vi "_interfacebrowser Build Status Menu.vi"(5 "Tree":refnum<vi>, 7 "CtlRef":refnum<vi>, 9 "Coords":T1, 11 "Menu in":refnum<k9>) -> (3 "Discard?":bool)   [LabVIEW 2017, in "interfacebrowser.lvlib"]
uses:
  interfacebrowser.lvlib
  <vilib>/Utility/miscctls.llb/LVPoint32TypeDef.ctl
  _csmHelper/API with lvcsm Support/CSM-Helper API with lvcsm Support.lvlib
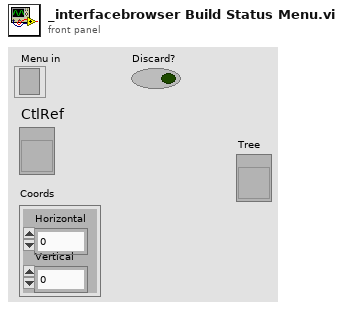
[diagram p1: front panel]
types:
  T1 = typedef "LVPoint32TypeDef.ctl" = cluster{"Horizontal":i32, "Vertical":i32}
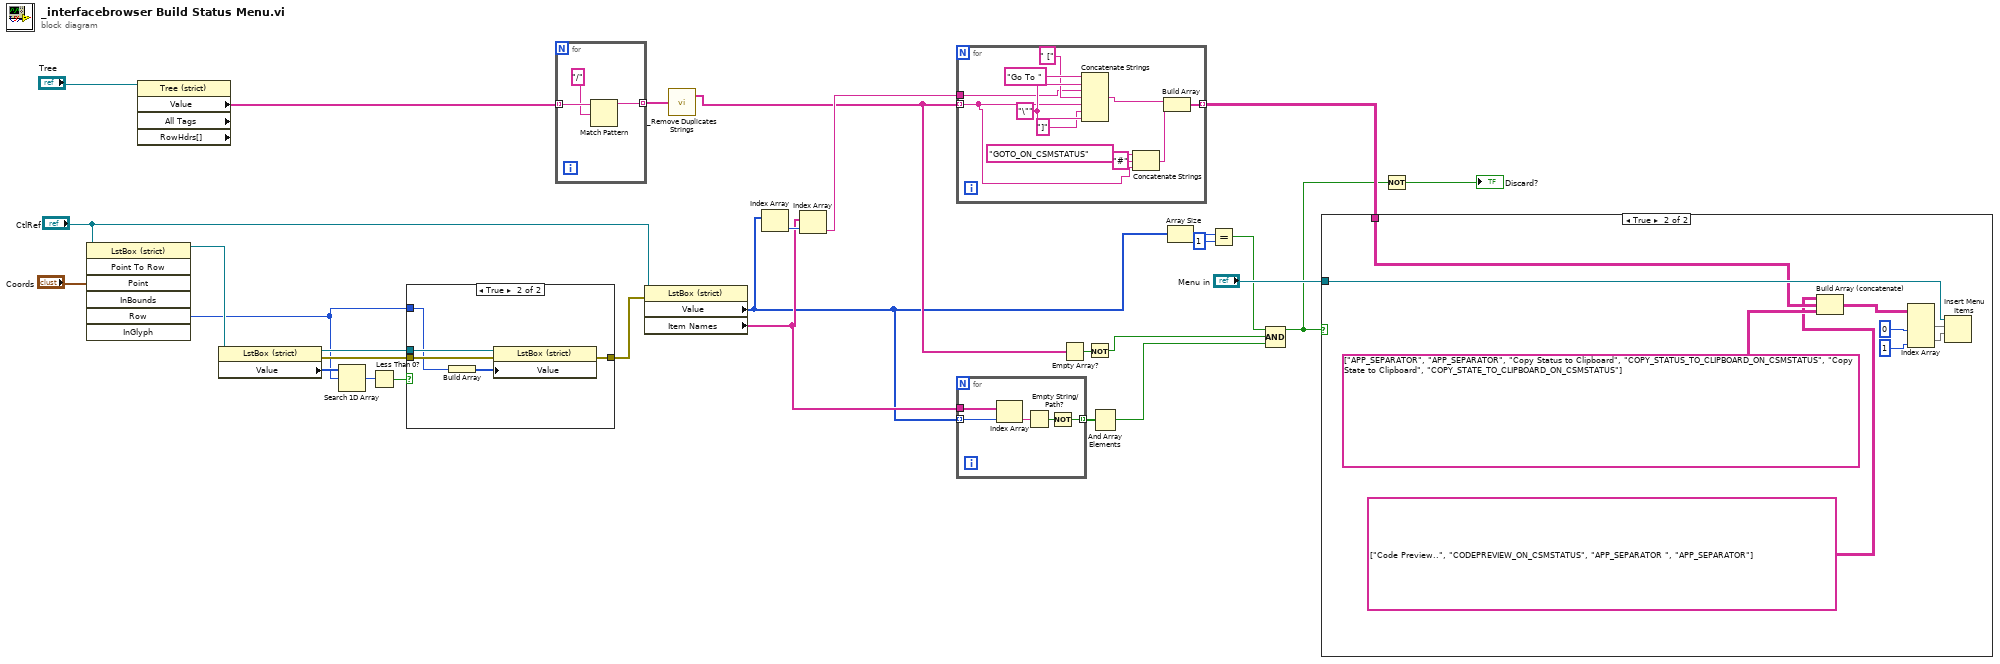
[diagram p0: block diagram]
diagram:
  n1 = invoke on="Invoke Node" class="LstBox (strict)" method="Point To Row"(reference="CtlRef", "Point"="Coords") -> (reference out=w26:refnum<vi>, "Row"=w19:i32)  [unwired: 5 in, 5 out]
  n2 = property on="Property Node" class="Tree (strict)" props=["Value", "All Tags", "RowHdrs[]"](reference="Tree") -> ("Value"=w14:string[])  [unwired: 1 in, 4 out]
  n3 = property on="Property Node" class="LstBox (strict)"(reference=w26) -> (reference out=w23:refnum<vi>, error out=w24:errorcluster, "Value"=w20:i32[])  [unwired: 1 in]
  n4 = Search 1D Array(1D array=w20, element=w19) -> (index of element=w25:i32)  [unwired: 1 in]
  n5 = Less Than 0?(x=w25) -> (x < 0?=w22:bool)
  n6 = case shown="True" w22 {
    tunnel: w24 -> [w30 w35]
    tunnel: w23 -> [_ w34]
    tunnel: w19 -> [_ w33]
    tunnel: [w30 w32] -> w21
    frame False {
    }
    frame True {
      n7 = Build Array(w33) -> (w31:i32[])
      n8 = property on="Property Node" class="LstBox (strict)"(reference=w34, error in=w35, "Value"=w31) -> (error out=w32:errorcluster)  [unwired: 1 out]
    }
  }
  n9 = for {
    tunnel: w14 -> [w38] mode=indexing
    tunnel: [w36] -> w13 mode=indexing
    n10 = Match Pattern(string=w38, regular expression="/") -> (before substring=w36:string)  [unwired: 1 in, 3 out]
  }
  n11 = property on="Property Node" class="LstBox (strict)"(reference="CtlRef", error in=w21) -> ("Value"=w9:i32[], "Item Names"=w10:string[])  [unwired: 2 out]
  n12 = call "_Remove Duplicates Strings.vi"("Input Array"=w13) -> ("Output Array"=w12:string[])  [unwired: 1 out]
  n13 = Index Array(array=w9) -> (element=w16:i32)  [unwired: 1 in]
  n14 = Index Array(array=w10, index=w16) -> (element=w15:string)
  n15 = for {
    tunnel: w12 -> [w40] mode=indexing
    tunnel: [w45] -> w17 mode=indexing
    tunnel: w15 -> [w43]
    w48 = "\"" ("string")
    n16 = Concatenate Strings("Go To " ("string"), w48, w43, " [" ("string"), w40, "]" ("string"), w48) -> (w47:string)
    n17 = Concatenate Strings("GOTO_ON_CSMSTATUS", "#" ("string"), w40) -> (w42:string)
    n18 = Build Array(w47, w42) -> (w45:string[])
  }
  n19 = for {
    tunnel: w10 -> [w54]
    tunnel: w9 -> [w53] mode=indexing
    tunnel: [w50] -> w8 mode=indexing
    n20 = Index Array(array=w54, index=w53) -> (element=w52:string)
    n21 = Empty String/Path?(string/path=w52) -> (empty?=w51:bool)
    n22 = Not(x=w51) -> (.not. x?=w50:bool)
  }
  n23 = Empty Array?(array=w12) -> (empty?=w11:bool)
  n24 = Not(x=w11) -> (.not. x?=w7:bool)
  n25 = And Array Elements(Boolean array=w8) -> (logical AND=w6:bool)
  n26 = Array Size(array=w9) -> (size(s)=w5:i32)
  n27 = Equal?(x=w5, y=1) -> (x = y?=w3:bool)
  n28 = Compound Arithmetic op=AND(w3, w7, w6) -> (w2:bool)
  n29 = case shown="True" w2 {
    tunnel: "Menu in" -> [_ w63]
    tunnel: w17 -> [_ w56]
    frame False {
    }
    frame True {
      n30 = Build Array (concatenate)(string[][] [["Code Preview..", "CODEPREVIEW_ON_CSMSTATUS"], ["APP_SEPARATOR ", "APP_SEPARATOR"]] ("item names"), w56, string[][] [["APP_SEPARATOR", "APP_SEPARATOR"], ["Copy Status to Clipboard", "COPY_STATUS_TO_CLIPBOARD_ON_CSMSTATUS"], ["Copy State to Clipboard", "COPY_STATE_TO_CLIPBOARD_ON_CSMSTATUS"]] ("item names")) -> (w57:string[][])
      n31 = Index Array(array=w57, index (col) #1=0 ("disabled index (col)"), index (col) #2=1 ("index (col)")) -> (element #1=w61:string[], element #2=w60:string[])  [unwired: 2 in]
      n32 = Insert Menu Items(7:w60, 8:w61, 9:w63) -> ()  [unwired: 3 in, 3 out]
    }
  }
  n33 = Not(x=w2) -> (.not. x?=→"Discard?":bool)
